vi "Voltage ch0-1_mean_ch2_pk-pk - Continuous Input.vi"() -> ()   [LabVIEW 2012]
doc: "This example demonstrates how to continuously acquire buffered voltage measurements using a DAQmx device. It uses software events to ensure that the program does not become unresponsive while waiting for samples to become available.\n\nFor instructions on how to connect your signals to the DAQ device, refer to your device documentation."
uses:
  <vilib>/DAQmx/read.llb/DAQmx Read (Analog 1D Wfm NChan NSamp).vi
  <vilib>/DAQmx/create/channels.llb/DAQmx Create Channel (AI-Voltage-Basic).vi
  <vilib>/DAQmx/configure/timing.llb/DAQmx Timing (Sample Clock).vi
  <vilib>/DAQmx/configure/task.llb/DAQmx Configure Logging (TDMS).vi
  <vilib>/DAQmx/miscellaneous.llb/DAQmx Fill In Error Info.vi
  <resource>/objmgr/daqmx.rc
panel:
  out "Ch2 Pk-pk DC(V)":string
  out "Ch0 Mean DC (V)":string
  out "Ch1 Mean DC (V)":string
  in  "File Name and Path File Root Name":path
  in  "Stop":bool
  out "Waveform Graph":waveform(dbl)[](graph)
  in  "Samples per Loop":i32=50000
  in  "Sample Rate":dbl=50000.0
  in  "Sample Clock Source":tag="OnboardClock"
  in  "Terminal Configuration":i32(ring)=-1 items=["default"=-1, "RSE"=10083, "NRSE"=10078, "Differential"=10106, "Pseudodifferential"=12529]
  in  "Max Voltage":dbl=5.0
  in  "Min Voltage":dbl=-5.0
  in  "Physical Channel":tag="Dev1/ai0:2"
  out "Actual Sample Rate":dbl format="%0.2f"
  # "Channel Settings"
  # "Indicators"
  # "Acquired \"Raw\" Data"
  # "Timing Settings"
  # "Logging Settings"
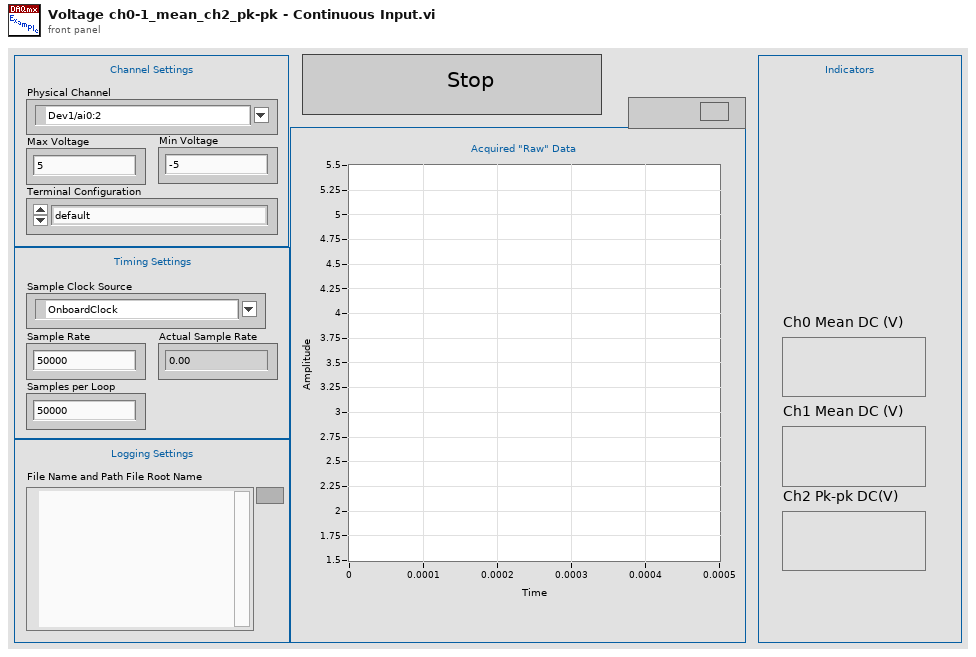
[diagram p1: front panel]
types:
  T1 = enum16{"open", "replace", "create", "open or create", "replace or create", "replace or create with confirmation"}
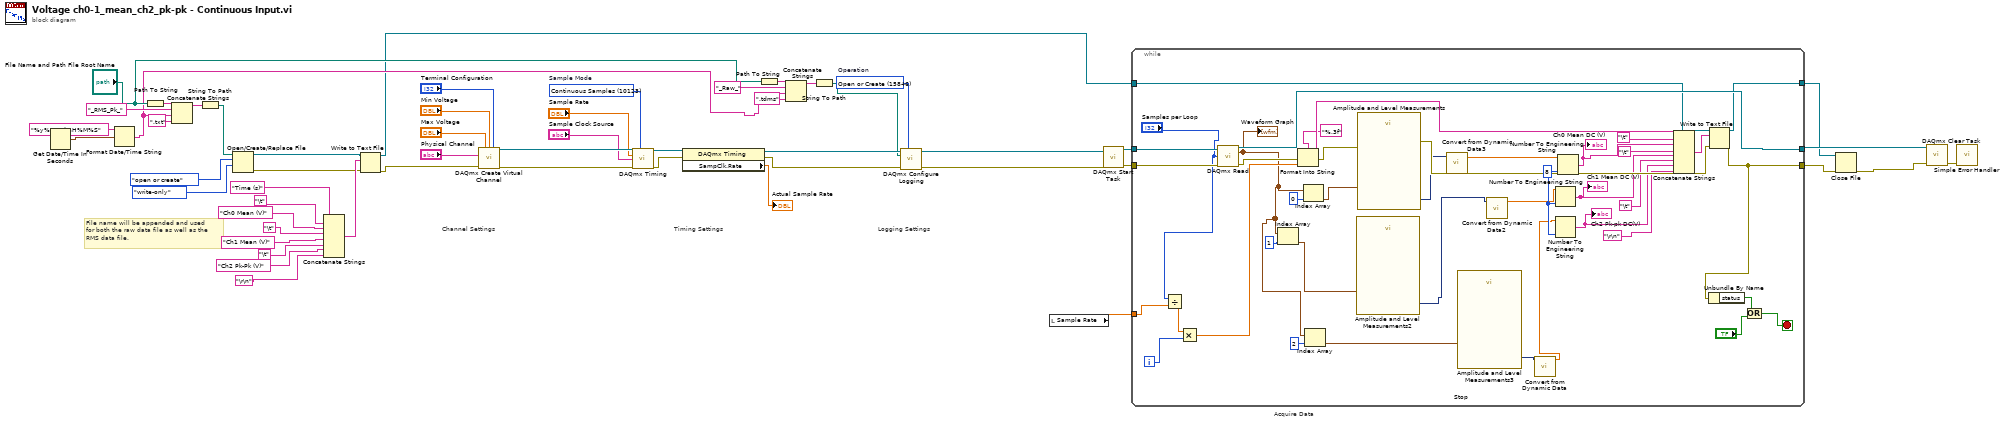
[diagram p0: block diagram]
diagram:
  w47 = 15846 items=["Open"=10437, "Open or Create"=15846, "Create or Replace"=15847, "Create"=15848]  # Operation
  w52 = 10123 items=["Finite Samples"=10178, "Continuous Samples"=10123, "Hardware Timed Single Point"=12522]  # Sample Mode
  # "File name will be appended and used\nfor both the raw data file as well as the \nRMS data file."
  # "Acquire Data"
  # "Logging Settings"
  # "Timing Settings"
  # "Channel Settings"
  n1 = Get Date/Time In Seconds() -> (seconds since 1Jan1904=w24:timestamp)
  n2 = Format Date/Time String(time format string (%c)="%y%m%d%H%M%S", seconds (now)=w24) -> (date/time string=w14:string)  [unwired: 1 in]
  n3 = Path To String(path="File Name and Path File Root Name") -> (string=w27:string)
  n4 = Concatenate Strings(w27, "_RMS_Pk_" ("string"), w14, ".txt" ("string")) -> (w26:string)
  n5 = String To Path(string=w26) -> (path=w25:path)
  n6 = Open/Create/Replace File(file path (use dialog)=w25, operation (0:open)=T1."open or create", access (0:read/write)=enum16{"read/write", "read-only", "write-only"}."write-only") -> (refnum out=w3:refnum<file>, error out=w5:errorcluster)  [unwired: 1 in, 3 out]
  n7 = Concatenate Strings("Time (s)" ("RMS (V) 2"), "\t", "Ch0 Mean (V)" ("RMS (V) 2"), "\t", "Ch1 Mean (V)" ("Peak-to-Peak (V) 2"), "\t", "Ch2 Pk-Pk (V)" ("Mean DC (V) 2"), "\r\n") -> (w10:string)
  n8 = Write to Text File(file (use dialog)=w3, text=w10, error in=w5) -> (refnum out=w2:refnum<file>, error out=w4:errorcluster)  [unwired: 1 in, 1 out]
  n9 = call-poly <vilib>:"DAQmx Create Virtual Channel.vi"("maximum value"="Max Voltage", "minimum value"="Min Voltage", "input terminal configuration"="Terminal Configuration", "physical channels"="Physical Channel", "error in"=w4) -> ("task out"=w50:refnum<k21>, "error out"=w51:errorcluster)  [unwired: 9 in]
  n10 = call-poly <vilib>:"DAQmx Timing.vi"("task/channels in"=w50, "sample mode"=w52, "rate"="Sample Rate", "source"="Sample Clock Source", "error in"=w51) -> ("task out"=w54:refnum<k21>, "error out"=w53:errorcluster)  [unwired: 9 in]
  n11 = property class="DAQmx Timing"(reference=w54, error in=w53) -> (reference out=w49:refnum<k21>, error out=w48:errorcluster, "SampClk.Rate"=→"Actual Sample Rate":dbl)
  n12 = Path To String(path="File Name and Path File Root Name") -> (string=w17:string)
  n13 = Concatenate Strings(w17, "_Raw_" ("string"), w14, ".tdms" ("string")) -> (w18:string)
  n14 = String To Path(string=w18) -> (path=w16:path)
  n15 = call-poly <vilib>:"DAQmx Configure Logging.vi"("task/channels in"=w49, "operation"=w47, "file path"=w16, "error in"=w48) -> ("task out"=w30:refnum<k21>, "error out"=w29:errorcluster)  [unwired: 10 in]
  n16 = local read "Sample Rate"() -> (w33:dbl)
  n17 = call <vilib>:"DAQmx Start Task.vi"("task/channels in"=w30, "error in"=w29) -> ("task out"=w37:refnum<k21>, "error out"=w38:errorcluster)  [unwired: 12 in]
  n18 = while {
    tunnel: w38 -> [w95]
    tunnel: w37 -> [w94]
    tunnel: [w93] -> w36
    tunnel: [w78] -> w32
    tunnel: w33 -> [w91]
    tunnel: w2 -> [w90]
    tunnel: [w89] -> w31
    i -> [w92]
    stop <- w75 stop-if-true
    w71 = i16 8 ("precision (6)")
    n19 = Divide(x="Samples per Loop", y=w91) -> (x/y=w88:dbl)
    n20 = Multiply(x=w88, y=w92) -> (x*y=w87:dbl)
    n21 = call-poly <vilib>:"DAQmx Read.vi"("task/channels in"=w94, "number of samples per channel"="Samples per Loop", "error in"=w95) -> ("task out"=w93:refnum<k21>, "data"=w58:waveform(dbl)[], "error out"=w86:errorcluster)  [unwired: 10 in]
    "Waveform Graph" <- w58
    n22 = Index Array(array=w58, index=1) -> (element=w61:waveform(dbl))
    n23 = Format Into String(format string="%.3f", error in=w86, w87) -> (resulting string=w84:string, error out=w82:errorcluster)  [unwired: 1 in]
    n24 = Index Array(array=w58, index=0) -> (element=w66:waveform(dbl))
    n25 = Index Array(array=w58, index=2) -> (element=w57:waveform(dbl))
    n26 = call "Amplitude and Level Measurements2"("Signals"=w61) -> ("Mean (DC)"=w60:dynamicdata)  [unwired: 9 in, 5 out]
    n27 = call "Amplitude and Level Measurements"("Signals"=w66, "error in (no error)"=w82) -> ("Mean (DC)"=w70:dynamicdata, "error out"=w81:errorcluster)  [unwired: 8 in, 4 out]
    n28 = call "Convert from Dynamic Data3"("Dynamic Data Type"=w70) -> ("Scalar"=w65:dbl)  [unwired: 3 in]
    n29 = call "Amplitude and Level Measurements3"("Signals"=w57) -> ("Peak to Peak"=w56:dynamicdata)  [unwired: 9 in, 5 out]
    n30 = call "Convert from Dynamic Data2"("Dynamic Data Type"=w60) -> ("Scalar"=w80:dbl)  [unwired: 3 in]
    n31 = call "Convert from Dynamic Data"("Dynamic Data Type"=w56) -> ("Scalar"=w55:dbl)  [unwired: 3 in]
    n32 = Number To Engineering String(2:w71, 4:w80) -> (0:w64:string)  [unwired: 2 in]
    "Ch1 Mean DC (V)" <- w64
    n33 = Number To Engineering String(2:w71, 4:w55) -> (0:w63:string)  [unwired: 2 in]
    "Ch2 Pk-pk DC(V)" <- w63
    n34 = Number To Engineering String(2:w71, 4:w65) -> (0:w69:string)  [unwired: 2 in]
    "Ch0 Mean DC (V)" <- w69
    n35 = Concatenate Strings(w84, "\t", w69, "\t", w64, "\t", w63, "\r\n") -> (w85:string)
    n36 = Write to Text File(file (use dialog)=w90, text=w85, error in=w81) -> (refnum out=w89:refnum<file>, error out=w78:errorcluster)  [unwired: 1 in, 1 out]
    n37 = Unbundle By Name(w78) -> ("status"=w77:bool)
    n38 = Or(x=w77, y="Stop") -> (x .or. y?=w75:bool)
  }
  n39 = Close File(refnum=w31, error in=w32) -> (error out=w28:errorcluster)  [unwired: 1 out]
  n40 = call <vilib>:"DAQmx Clear Task.vi"("task in"=w36, "error in"=w28) -> ("error out"=w46:errorcluster)  [unwired: 13 in]
  n41 = call <vilib>:"Simple Error Handler.vi"("error in (no error)"=w46) -> ()  [unwired: 4 in, 5 out]
